vi "Configure Video Trigger.vi"(8 "error in (no error)":errorcluster {"code" format="%.0x"}, 9 "video trigger slope (Positive)":i32(ring)=1 items=["Positive"=1, "Negative"=2], 10 "video trigger level":dbl, 11 "instrument handle":refnum<k15>) -> (0 "error out":errorcluster {"code" format="%.0x"}, 3 "instrument handle out":refnum<k15>)   [LabVIEW 2009, in "Keysight XSAn.lvlib"]
doc: "This VI specifies the video level and slope for triggering.\n\nSupported Models: All supported"
uses:
  <instrlib>/Keysight XSAn/Keysight XSAn.lvlib
  AgXSAn.dll
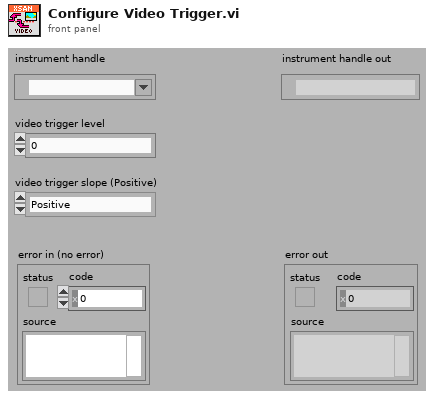
[diagram p1: front panel]
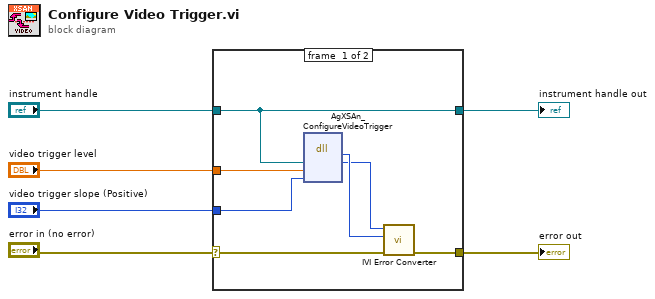
[diagram p0: block diagram]
diagram:
  n1 = case shown="No Error" "error in (no error)" {
    selector: "error in (no error)" -> [w12 w15]
    tunnel: [w13 w15] -> w5
    tunnel: "instrument handle" -> [w10 w14]
    tunnel: [w10 w14] -> w3
    tunnel: "video trigger level" -> [w9 _]
    tunnel: "video trigger slope (Positive)" -> [w8 _]
    frame #0 {
      n2 = dll-call lib="AgXSAn**.dll" fn="AgXSAn_ConfigureVideoTrigger" ("LabVIEW:IviSpecAn_ConfigureVideoTrigger")("instrument handle"=w10, "video trigger level"=w9, "video trigger slope"=w8) -> ("Status"=w11:i32, "instrument handle"=w7:u32)  [unwired: 5 in, 2 out]
      n3 = call <instrlib>:"IVI Error Converter.vi"("error in (no error)"=w12, "IVI error code (0)"=w11, "instrument handle"=w7) -> ("error out"=w13:errorcluster)  [unwired: 7 in, 1 out]
    }
    frame #1 {
    }
  }
  "error out" <- w5
  "instrument handle out" <- w3
